vi "Measurements.vi"(8 "error in (no error)":errorcluster, 11 "Configuration in":refnum<class "Configuration.lvclass">) -> (0 "error out":errorcluster, 3 "Configuration out":refnum<class "Configuration.lvclass">)   [LabVIEW 2026, in "Msmt Configuration.lvlib" / "Controller Configuration.lvclass"]
uses:
  Controller Configuration.lvclass
  configuration/Configuration.lvclass
  C:/Users/E2013170/Documents/GitHub/Measurement-Utility-Reference/source/configuration/Configuration.lvclass
  Controller Configuration.lvclass/Controller Configuration.ctl
panel:
  in  "Load Msmts from Application Data Directory":bool
  in  "Paths to Load Measurements From":i32(listbox)
  in  "Delete":bool
  in  "Add":bool
  # "Specify additional paths to load measurement plugins from:"
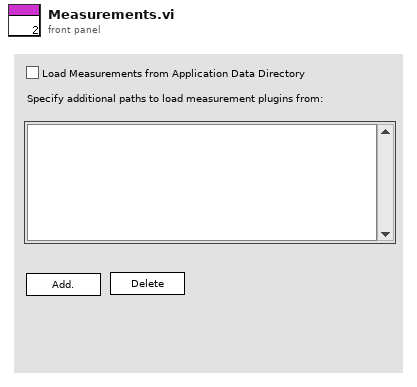
[diagram p1: front panel]
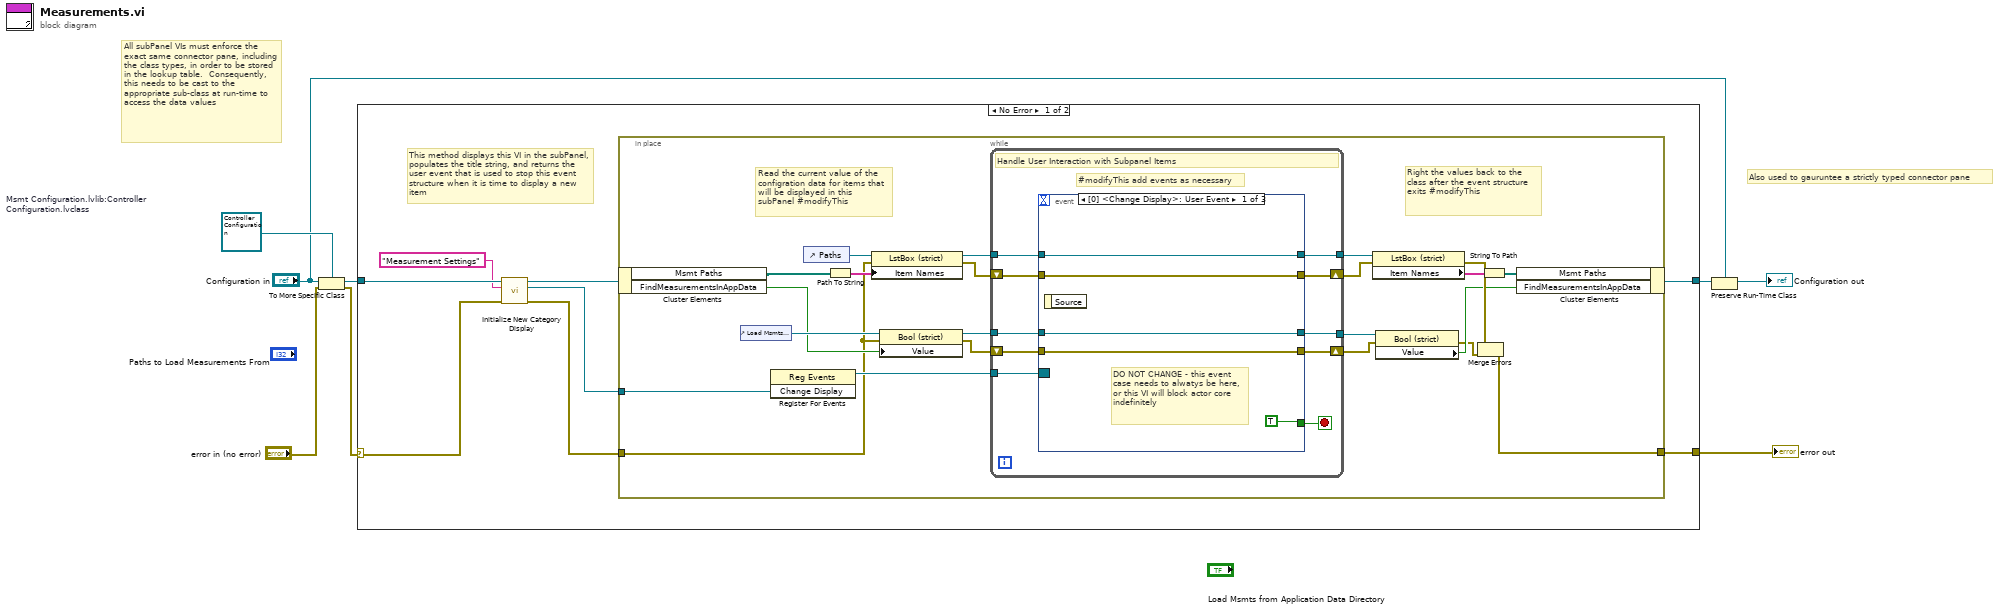
[diagram p0: block diagram]
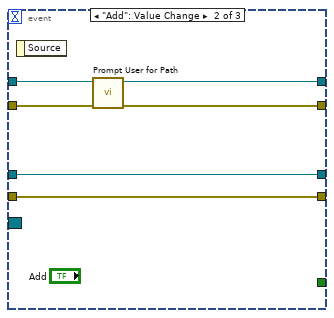
[diagram p2: hidden frame]
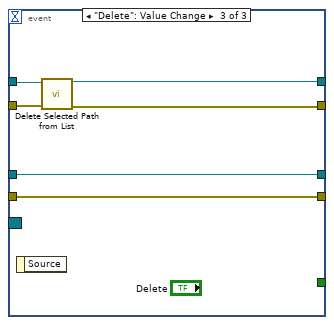
[diagram p3: hidden frame]
diagram:
  w5 = refnum<class "Controller Configuration.lvclass"> refnum  # Msmt Configuration.lvlib:Controller Configuration.lvclass
  # "Also used to gauruntee a strictly typed connector pane"
  # "All subPanel VIs must enforce the exact same connector pane, including the class types, in order to be stored in the lookup table.  Consequently, this needs to be cast to the appropriate sub-class at run-time to access the data values"
  n1 = To More Specific Class(target class=w5, reference="Configuration in", error in="error in (no error)") -> (specific class reference=w6:refnum<class "Controller Configuration.lvclass">, error out=w1:errorcluster)
  n2 = case shown="No Error" w1 {
    selector: w1 -> [w10 w66]
    tunnel: w6 -> [w16 w67]
    tunnel: [w14 w67] -> w8
    tunnel: [w12 w66] -> w7
    frame No Error {
      # "This method displays this VI in the subPanel, populates the title string, and returns the user event that is used to stop this event structure when it is time to display a new item"
      n3 = call "Initialize New Category Display.vi"("error in (no error)"=w10, "Name to Display"="Measurement Settings", "Configuration in"=w16) -> ("error out"=w13:errorcluster, "Change Display"=w9:refnum<user-event>, "Configuration Out"=w15:refnum<class "Controller Configuration.lvclass">)  [unwired: 6 in]
      n4 = in-place {
        in-place-border: w13 -> [w24]
        in-place-border: [w20] -> w12
        in-place-border: w9 -> [w33]
        # "Right the values back to the class after the event structure exits #modifyThis"
        # "Read the current value of the configration data for items that will be displayed in this subPanel #modifyThis"
        n5 = in-place-cluster #1(w15) -> ("Msmt Paths"=w37:path[], "FindMeasurementsInAppData"=w25:bool)
        n6 = control-ref of="Load Msmts from Application Data Directory"() -> (w26:refnum<vi>)
        n7 = register-events(w33) -> (reference out=w32:refnum<event-registration>)  [unwired: 2 in, 1 out]
        n8 = control-ref of="Paths"() -> (w29:refnum<vi>)
        n9 = Path To String(path=w37) -> (string=w38:string[])
        n10 = property on="Property Node" class="LstBox (strict)"(reference=w29, error in=w24, "Item Names"=w38) -> (reference out=w28:refnum<vi>, error out=w31:errorcluster)
        n11 = property on="Property Node" class="Bool (strict)"(reference=w26, error in=w24, "Value"=w25) -> (reference out=w23:refnum<vi>, error out=w18:errorcluster)
        n12 = while {
          tunnel: w32 -> [w47]
          shift-right: [w46] -> w30
          shift-left: w31 -> [w43]
          tunnel: w28 -> [w45]
          tunnel: [w44] -> w27
          tunnel: [w42] -> w22
          tunnel: w23 -> [w41]
          shift-right: [w39] -> w17
          shift-left: w18 -> [w40]
          stop <- w48 stop-if-true
          # "#modifyThis add events as necessary"
          # "Handle User Interaction with Subpanel Items"
          n13 = event shown="[0] <Change Display>: User Event" {
            selector: w47 -> [_ _ _]
            dyn-events: _ -> [_ _ _]
            timeout: _ -> [_ _ _]
            tunnel: [TRUE _ _] -> w48
            tunnel: [w51 w57 w63] -> w46
            tunnel: w45 -> [w52 w59 w65]
            tunnel: [w52 w56 w62] -> w44
            tunnel: w43 -> [w51 w58 w64]
            tunnel: [w50 w55 w61] -> w42
            tunnel: w41 -> [w50 w55 w61]
            tunnel: w40 -> [w49 w54 w60]
            tunnel: [w49 w54 w60] -> w39
            event User Event {
              # "DO NOT CHANGE - this event case needs to alwatys be here, or this VI will block actor core indefinitely"
              n14 = event-data() -> ()  [unwired: 1 in, 1 out]
            }
            event "Add": Value Change {
              n15 = event-data() -> ()  [unwired: 1 in, 1 out]
              n16 = call "Prompt User for Path.vi"("error in (no error)"=w58, "ListBox in"=w59) -> ("error out"=w57:errorcluster, "ListBox out"=w56:refnum<vi>)  [unwired: 8 in]
            }
            event "Delete": Value Change {
              n17 = event-data() -> ()  [unwired: 1 in, 1 out]
              n18 = call "Delete Selected Path from List.vi"("error in (no error)"=w64, "ListBox in"=w65) -> ("error out"=w63:errorcluster, "ListBox out"=w62:refnum<vi>)  [unwired: 8 in]
            }
          }
        }
        n19 = property on="Property Node" class="LstBox (strict)"(reference=w27, error in=w30) -> (error out=w34:errorcluster, "Item Names"=w36:string[])  [unwired: 1 out]
        n20 = property on="Property Node" class="Bool (strict)"(reference=w22, error in=w17) -> (error out=w19:errorcluster, "Value"=w21:bool)  [unwired: 1 out]
        n21 = Merge Errors(w34, w19) -> (w20:errorcluster)
        n22 = String To Path(string=w36) -> (path=w35:path[])
        n23 = in-place-cluster #1("Msmt Paths"=w35, "FindMeasurementsInAppData"=w21) -> (w14:refnum<class "Controller Configuration.lvclass">)
      }
    }
    frame Error {
    }
  }
  "error out" <- w7
  n24 = Preserve Run-Time Class(object in=w8, 2:"Configuration in") -> (object out=→"Configuration out":refnum<class "Configuration.lvclass">)  [unwired: 1 in, 1 out]
